vi "Report - Excel.vi"(4 "pdf":bool=TRUE, 5 "Chart Seperation by Order#":bool=TRUE, 6 "Details from .stp and Parameters":string="Transaction Run No\t15\r\nNo.\t1\r\nOrder No.\t105\r\nOper. No.\t1051\r\nQty.\t1052\r\nNCR No.\t1053\r\nCustomer Name\tCustomer 105\r\nProject\tProject 105\r\nSales Order\tSO105\r\nItem No.\tSO105\r\nMaterial\tM105\r\nMaterial Description\tM105 Description\r\nRevision\t\r\nSerial No.\t105\r\nTC1\t2\r\nTC2\t\r\nTC3\t\r\nTC4\t\r\nTC5\t\r\nTC6\t\r\nTC01Plot\t1\r\nTC02Plot\t0\r\nTC03Plot\t0\r\nTC04Plot\t0\r\nTC05Plot\t0\r\nTC06Plot\t0\r\nNotes\t\r\nPermitted Temp Diff\t4\r\nPermitted Time Diff\t30\r\nSequence Number\t1\t2\r\nRamp Rate\t150\t50\r\nTarget Temperature\t60\t40\r\nHold Time Duration\t00:20\t00:00\r\nName\tTemperature Controller\tTemperature Module\tTemperature Module\tTemperature Module\r\nModel\tET-3504\tNI-9211\tNI-9211\tNI-9211\r\nEquipment Serial No.\tE123-02\t12F0001\t12F0002\t12F0003\r\nLast Calibration Date\t2013-12-22\t2014-01-01\t2014-02-02\t2014-09-23\r\nNext Calibration Date\t2014-12-22\t2015-01-01\t2015-09-28\t2015-09-01\r\nEquipment ID\tET-3504 02\tNI-9211 01\tNI-9211 02\tNI-9211 03\r\nNotice Period\t30\t60\t0\t0\r\nWPS/Ref\tWPS2\r\nWPS Rev\t1\r\nHold Temperature\t60\r\nWPS Details Temperature Units\t°C\r\nHold Time (HH:MM)\t00:20\r\nExtra WPS\tWPS2\r\nExtra Rev\t1\r\nAdditional WPS Number\t,\r\nOutput Set\t001\r\nFurnace Serial No\tA1234A1\r\nLast Inspection Date\t2013-12-22\r\nNext Inspection Due Date\t2014-12-22\r\nChannel to Probe Mapping\t1,2,3,4,5,6,7,8,9,10,11,12,13,14,15,16\r\n[StartRecordTime]\t2014-12-02 08:49:30\r\n[StartRecordTemp]\t27.62\r\n[MaxRecordedTemp]\t60.3\r\n[MaxRecordedTempTime]\t2014-12-02 09:04:30\r\n[MinRecordedTemp]\t27.62\r\n[MinRecordedTempTime]\t2014-12-02 08:49:30\r\n[EndRecordTemp]\t37.15\r\n[EndRecordTime]\t2014-12-02 09:50:31\r\n[RecordedMinutes]\t61\r\n[StartHoldTime]\t2014-12-02 09:02:31\r\n[StartHoldTemp]\t60\r\n[HoldTimeMaxTemp]\t60.3\r\n[HoldTimeMinTemp]\t59.75\r\n[EndHoldTime]\t2014-12-02 09:22:31\r\n[EndHoldTemp]\t60\r\n[HoldDurationMinutes]\t0:20\r\n[TempDiffDuringHold]\t0.55\r\n[UnitOfTemperature]\t°C\r\n[PerformedBy]\tadmin\r\n[PerformedOn]\t2014-12-02 08:49:30\r\n[IsTempWithinTol]\t-1\r\n[IsTimeWithinTol]\t-1\r\n[ProcessStatus]\t1\r\n[OverallStatus]\t1\r\n[Result]\t1\r\n[RawDataFilePath]\tc:\\temp\\SRTRS4070_Host\\Data_Host\\2014\\12\\\r\n[RawDataFileName]\t147_20141202_084930.dat\r\n[SavedBy]\tadmin\r\nUsername\tAdministrator\r\n", 7 "Use DB for Picture (Material)":bool=TRUE, 8 "error in (no error)":errorcluster, 9 "Include MetaData":bool=TRUE, 10 "Report Additional Details":T1, 11 "Report Files Cluster":T2) -> (0 "error out":errorcluster, 1 "Picture Error":errorcluster, 2 "Material File":string)   [LabVIEW 2013]
uses:
  Controls/Report Files Cluster.ctl
  Controls/Report Additional Details Cluster.ctl
  Controls/DB - Master Data Material Enum.ctl
  Controls/DB - OpenClose.ctl
  <vilib>/Utility/NIReport.llb/NI_report.lvclass
  <vilib>/Utility/file.llb/Read From Spreadsheet File (string).vi
  Controls/Global SRTRS.vi
  <vilib>/addons/_office/excel.llb/Excel Easy Table (str).vi
  <vilib>/Utility/NIReport.llb/Excel/NI_Excel.lvclass
  <vilib>/addons/_office/NI_ReportGenerationToolkit.lvlib
panel:
  out "DB Error":errorcluster
  in  "Close Excel":bool=TRUE
  in  "Include ConvFromUnicode":bool
  in  "Material":T3
  out "Reference Error Out":errorcluster
  out "Shape Name":string
  out "Order No Data from .dat File":string[][](array[string])
  out "Year":string
  out "Details from .stp and Parameters":string[][](array[string])=[["No.", "2", "", ""], ["Order No.", "123456002", "", ""], ["Operation No.", "202", "", ""], ["Qty (EA)", "201", "", ""], ["NCR No.", "203", "", ""], ["Customer", "Customer 204", "", ""], ["Project", "205", "", ""], ["Sales Order No.", "206", "", ""], ["Item No.", "207", "", ""], ["Material", "102-04", "", ""], ["BOM Rev.", "5", "", ""], ["Material Description", "Mat5", "", ""], ["Serial No.", "208", "", ""], ["TC1", "", "", ""], ["TC2", "", "", ""], ["TC3", "", "", ""], ["TC4", "4", "", ""], ["TC5", "5", "", ""], ["TC6", "6", "", ""], ["Notes", "Notes 200", "", ""], ["User", "Admin", "", ""], ["Customer No.", "", "", ""], ["Sequence Number", "1", "2", ""], ["Ramp Rate (DegC / hour)", "100", "200", ""], ["Target Temperature (DegC)", "200", "400", ""], ["Additional WPS/Ref.", "MyWPS2", "", ""], ["Rev.", "1A", "", ""], ["Module Serial No.", "A12345", "B67890", ""], ["Calibration Date", "2013-11-01", "2013-11-15", ""], ["Calibration Due", "2014-11-01", "2014-11-15", ""], ["WPS/Ref", "MyWPS", "", ""], ["Rev", "1C", "", ""], ["Hold Temperature", "500", "", ""], ["WPS Details Temperature Units", "", "", ""], ["Hold Time (HH:MM)", "4:00", "", ""], ["Furnace Serial No", "100", "", ""], ["Survey Date", "2013-12-05", "", ""], ["Survey Due", "2014-12-05", "", ""]]
  out "pdf file":string="c:\\temp\\SRTRS4070\\Reports\\2013\\0090300212_123456002_20131223_231711.pdf"
  out "abcd.xls":string="0090300212_123456002_20131223_231711.xls"
  out "Month":string="2013"
  out "All Data from .dat File":string[][](array[string])=[["Time", "TC1", "TC2", "TC3", "TC4", "TC5", "TC6", "TC7", "TC8"], ["0", "6.3", "7.3", "7.3", "7.3", "7.3", "7.3", "7.3", "7.3"], ["1", "9.8", "10.8", "10.8", "10.8", "10.8", "10.8", "10.8", "10.8"], ["2", "14.0", "15.0", "15.0", "15.0", "15.0", "15.0", "15.0", "15.0"], ["3", "19.0", "20.0", "20.0", "20.0", "20.0", "20.0", "20.0", "20.0"], ["4", "24.7", "25.7", "25.7", "25.7", "25.7", "25.7", "25.7", "25.7"], ["5", "31.1", "32.1", "32.1", "32.1", "32.1", "32.1", "32.1", "32.1"], ["6", "38.2", "39.2", "39.2", "39.2", "39.2", "39.2", "39.2", "39.2"], ["7", "45.9", "46.9", "46.9", "46.9", "46.9", "46.9", "46.9", "46.9"], ["8", "54.2", "55.2", "55.2", "55.2", "55.2", "55.2", "55.2", "55.2"], ["9", "63.1", "64.1", "64.1", "64.1", "64.1", "64.1", "64.1", "64.1"], ["10", "72.5", "73.5", "73.5", "73.5", "73.5", "73.5", "73.5", "73.5"], ["11", "82.4", "83.4", "83.4", "83.4", "83.4", "83.4", "83.4", "83.4"], ["12", "92.8", "93.8", "93.8", "93.8", "93.8", "93.8", "93.8", "93.8"], ["13", "103.6", "104.7", "104.6", "104.6", "104.7", "104.6", "104.7", "104.6"], ["14", "114.8", "115.8", "115.8", "115.8", "115.8", "115.8", "115.8", "115.8"], ["15", "126.4", "127.4", "127.4", "127.4", "127.4", "127.4", "127.4", "127.4"], ["16", "138.2", "139.2", "139.2", "139.2", "139.2", "139.2", "139.2", "139.2"], ["17", "150.3", "151.3", "151.3", "151.3", "151.3", "151.3", "151.3", "151.3"], ["18", "162.5", "163.5", "163.5", "163.5", "163.5", "163.5", "163.5", "163.5"], ["19", "174.9", "175.9", "175.9", "175.9", "175.9", "175.9", "175.9", "175.9"], ["20", "187.4", "188.4", "188.4", "188.4", "188.4", "188.4", "188.4", "188.4"], ["21", "200.0", "201.0", "201.0", "201.0", "201.0", "201.0", "201.0", "201.0"], ["22", "212.6", "213.6", "213.6", "213.6", "213.6", "213.6", "213.6", "213.6"], ["23", "225.1", "226.1", "226.1", "226.1", "226.1", "226.1", "226.1", "226.1"], ["24", "237.5", "238.5", "238.5", "238.5", "238.5", "238.5", "238.5", "238.5"], ["25", "249.7", "250.7", "250.7", "250.7", "250.7", "250.7", "250.7", "250.7"], ["26", "261.8", "262.8", "262.8", "262.8", "262.8", "262.8", "262.8", "262.8"], ["27", "273.6", "274.6", "274.6", "274.6", "274.6", "274.6", "274.6", "274.6"], ["28", "285.2", "286.2", "286.2", "286.2", "286.2", "286.2", "286.2", "286.2"], ["29", "296.4", "297.3", "297.4", "297.3", "297.4", "297.4", "297.4", "297.3"]]
  # "2014-09-28 19:23"
  # "Transaction No,93\nNo.,2\nOrder No.,102\nOper. No.,102\nQty.,1\nNCR No.,102\nCustomer Name,Cust102\nProject,Proj102\nSales Order,SO102\nItem No.,SOI102\nMaterial,M102\nMaterial Description,Blue Arrow\nRevision,1\nSerial No.,102\nTC1,3\nTC2,4\nTC3,\nTC4,\nTC5,\nTC6,\nTC01Plot,1\nTC02Plot,1\nTC03Plot,0\nTC04Plot,0\nTC05Plot,0\nTC06Plot,0\nNotes,\nSequence Number,1,2\nRamp Rate,200,100\nTarget Temperature,100,25\nHold Time Duration,00:10,00:00\nModule Serial No.,ET-3504,NI-9211,NI-9211,NI-9211\nLast Calibration Date,E12345,12F0531,13C7150,A12345\nNext Calibration Date,2012-11-22,2014-01-01,2014-02-02,2014-09-23\n,2014-11-22,2015-01-01,2015-09-28,2015-09-01\nWPS5\n10\n100\n\n00:10\nWPS5\n10\nFurnace Serial No,A123456\nLast Inspection Date,2012-11-22\nNext Inspection Due Date,2014-11-22\nChannel to Probe Mapping,1,2,3,4,5,6,7,8,9,10,11,12,13,14,15,16\n[StartRecordTime],2014-09-28 19:41:56\n[StartRecordTemp],28.49\n[MaxRecordedTemp],\n[MaxRecordedTempTime],\n[MinRecordedTemp],\n[MinRecordedTempTime],\n[EndRecordTemp],24.89\n[EndRecordTime],2014-09-28 19:43:15\n[RecordedMinutes],-1\n[StartHoldTime],2014-09-28 19:42:18\n[StartHoldTemp],100\n[EndHoldTime],2014-09-28 19:42:28\n[EndHoldTemp],100\n[HoldDurationMinutes],0:00\n[TempDiffDuringHold],-99.5\n[UnitOfTemperature],\n[PerformedBy],100001\n[PerformedOn],2014-09-28 19:41:56\n[IsTempWithinTol],-1\n[IsTimeWithinTol],-1\n[ProcessStatus],P\n[OverallStatus],\n[Result],\n[RawDataFile],\n[RawDataFilePath],c:\\temp\\SRTRS4070_Host\\Data_Host\\2014\\09\n[RawDataFileName],93_20140928_194156.dat"
  # "Error -2146827284\nPossible Causes. \nMicrosoft Excel Refuse to accept ActiveX Client Request\nSolution: \nGoto Task Manager and End Task. \nOr Run cmd line End Task in LabVIEW code"
  # "Error -2146827284\nPossible Causes. \nFile cannot be created\nSolution: \nCheck Access rights to folder"
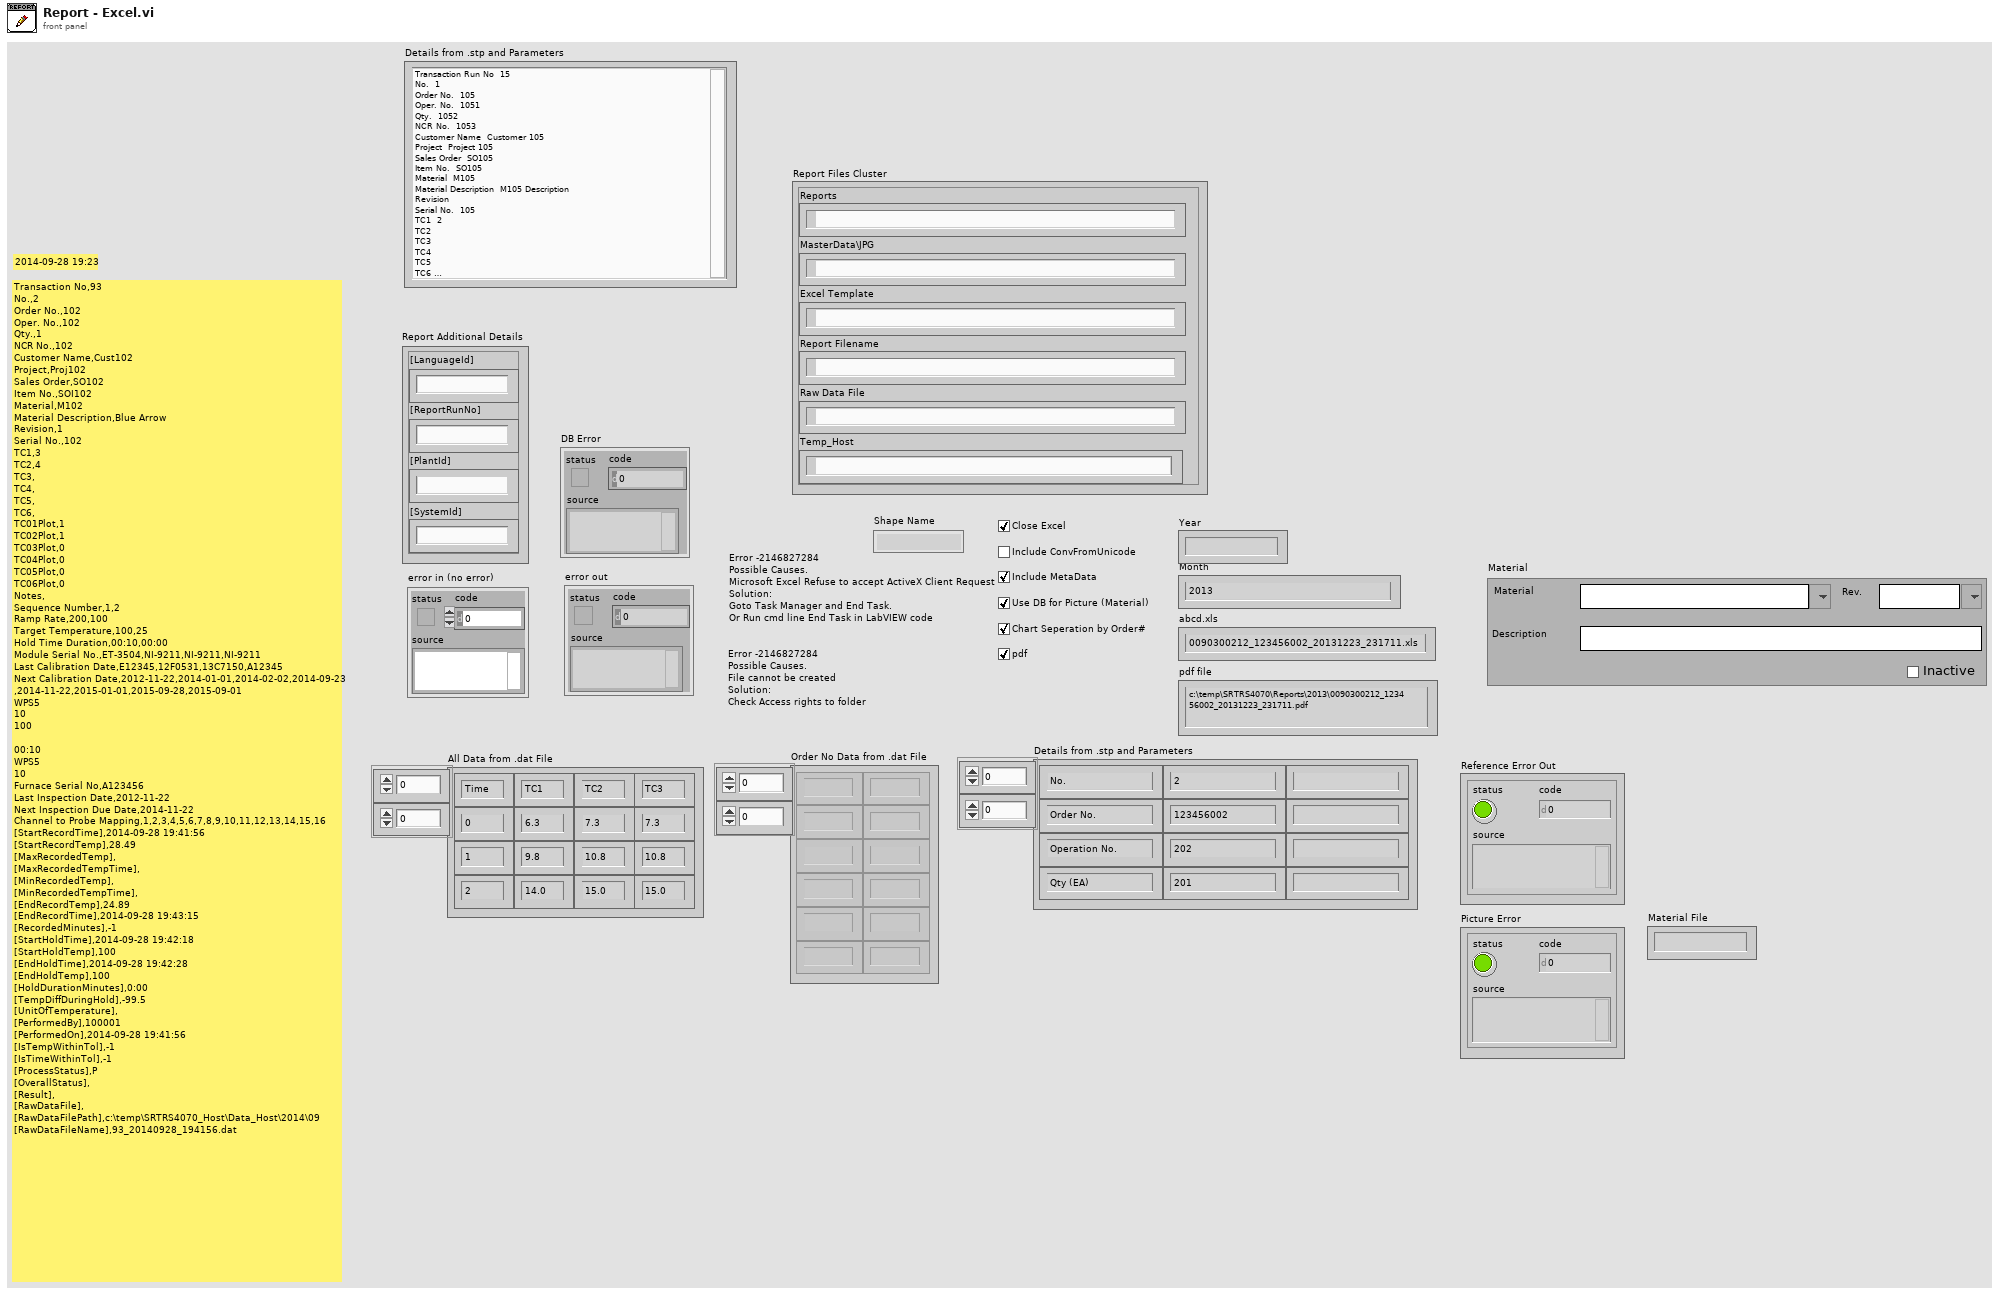
[diagram p1: front panel]
types:
  T1 = typedef "Report Additional Details Cluster.ctl" = cluster{"[LanguageId]":string, "[ReportRunNo]":string, "[PlantId]":string, "[SystemId]":string}
  T2 = typedef "Report Files Cluster.ctl" = cluster{"Reports":path, "MasterData\\JPG":path, "Excel Template":path, "Report Filename":path, "Raw Data File":path, "Temp_Host":path}
  T3 = cluster{"Master Data Material":string, "Master Data Rev":string, "Master Data Material Description":string, "Inactive":bool}
  T4 = cluster{"position (Excel)":cluster{"row":i32, "column":i32}, "name (Excel)":string, "bookmark (Word)":string}
  T5 = enum16{"maximized", "minimized", "normal", "no change"}
  T6 = enum16{"Standard Report", "HTML", "Word", "Excel"}
  T7 = typedef "DB - Logon Extra Info.ctl" = cluster{"Plant Name":string, "UserName":string, "Hostname [ClientName]":string, "IsUnicode":bool}
  T8 = typedef "DB - OpenClose.ctl" = cluster{"Open":bool, "Close":bool}
  T9 = typedef "DB - Master Data Material Enum.ctl" = enum16{"INSERT [MasterData].[Material]", "UPDATE [MasterData].[Material]", "SELECT [MaterialNo]", "SELECT [ShortDescription]", "SELECT [MaterialRev]", "SELECT [Description], [ImageFile]", "SELECT [Description] (Long)"}
  T10 = typedef "NI_Database_API.lvlib/Conn ObjectReference.ctl" = refnum<k1>
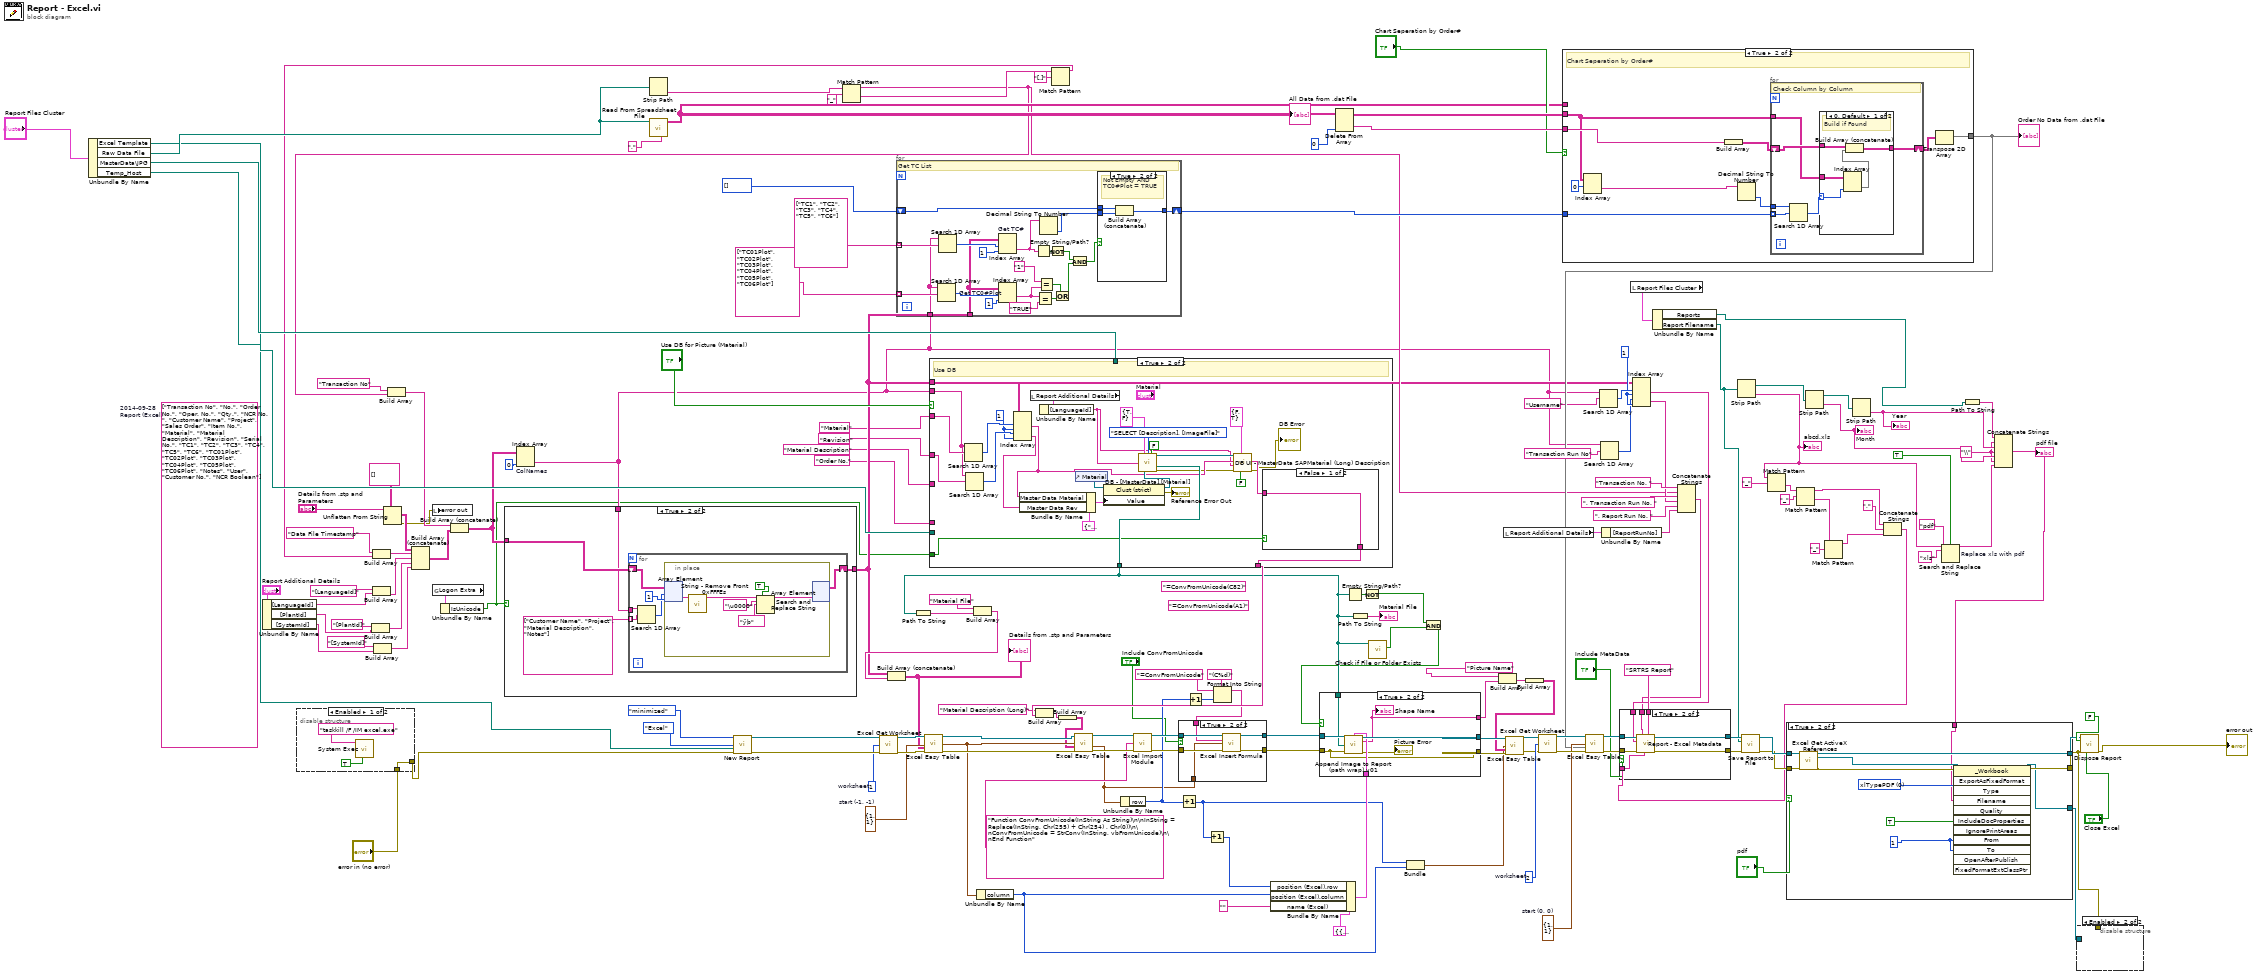
[diagram p0: block diagram]
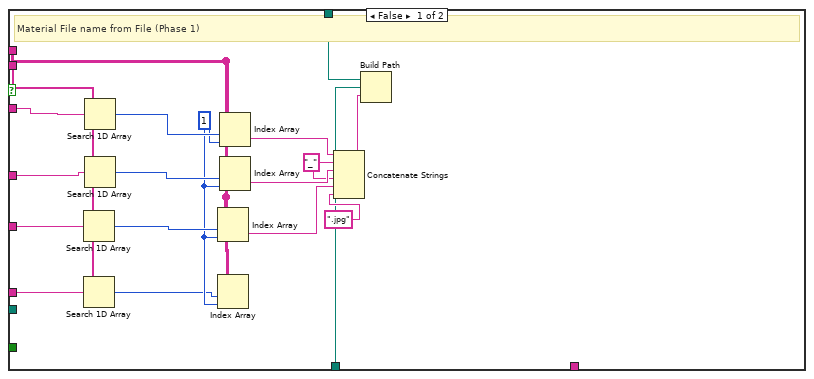
[diagram p5: hidden frame]
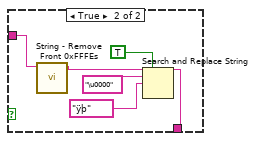
[diagram p6: hidden frame]
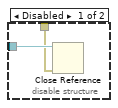
[diagram p11: hidden frame]
diagram:
  (unwired) "=ConvFromUnicode(C82)" ("text")
  (unwired) "=ConvFromUnicode(A1)" ("text")
  (unwired) string[] ["Transaction No", "No.", "Order No.", "Oper. No.", "Qty.", "NCR No.", "Customer Name", "Project", "Sales Order", "Item No.", "Material", "Material Description", "Revision", "Serial No.", "TC1", "TC2", "TC3", "TC4", "TC5", "TC6", "TC01Plot", "TC02Plot", "TC03Plot", "TC04Plot", "TC05Plot", "TC06Plot", "Notes", "User", "Customer No.", "NCR Boolean"]  # 2014-09-28 Report (Excel)
  w107 = 1 ("index (col)")
  w51 = "\\" ("string")
  w157 = cluster{"row":i32, "column":i32} {"row"=1, "column"=1}  # start (0, 0)
  w160 = 2  # worksheet
  w150 = cluster{"row":i32, "column":i32} {"row"=1, "column"=1}  # start (-1, -1)
  w162 = 1  # worksheet
  n1 = Unbundle By Name("Report Files Cluster") -> ("Excel Template"=w70:path, "Raw Data File"=w86:path, "MasterData\\JPG"=w82:path, "Temp_Host"=w81:path)
  n2 = Unbundle By Name("Report Additional Details") -> ("[LanguageId]"=w37:string, "[PlantId]"=w5:string, "[SystemId]"=w3:string)
  n3 = disable-structure shown="Enabled" {
    disable-tunnel: [w166 _] -> w142
    disable-tunnel: "error in (no error)" -> [w166 _]
    frame Enabled {
      n4 = call <vilib>:"System Exec.vi"("run minimized? (F)"=TRUE, "command line"="taskkill /F /IM excel.exe") -> ()  [unwired: 6 in, 4 out]
    }
    frame Disabled {
    }
  }
  n5 = Build Array("[PlantId]" ("string"), w5) -> (w2:string[])
  n6 = Build Array("[LanguageId]" ("string"), w37) -> (w35:string[])
  n7 = Build Array("[SystemId]" ("string"), w3) -> (w1:string[])
  n8 = Unflatten From String(type=string[][] [], binary string="Details from .stp and Parameters") -> (value=w41:string[][], error out=w13:errorcluster)  [unwired: 3 in, 1 out]
  n9 = local write "error out"(w13) -> ()
  n10 = global read "Global SRTRS.vi" "Logon Extra"() -> (w19:T7)
  n11 = Unbundle By Name(w19) -> ("IsUnicode"=w18:bool)
  n12 = Strip Path(path=w86) -> (name=w133:string)  [unwired: 1 out]
  n13 = call-poly <vilib>:"Read From Spreadsheet File.vi"("delimiter (\\t)"="," ("delimiter (\\t)"), "file path (dialog if empty)"=w86) -> ("all rows"=w100:string[][])  [unwired: 5 in, 4 out]
  "All Data from .dat File" <- w100
  n14 = call <vilib>:"New Report.vi"("window state (normal)"=T5."minimized", "report type"=T6."Excel", "template (empty)"=w70, "error in (no error)"=w142) -> ("report out"=w164:refnum<class "NI_report.lvclass">, "error out"=w163:errorcluster)  [unwired: 10 in]
  n15 = Match Pattern(string=w133, regular expression="_") -> (before substring=w33:string, after substring=w131:string)  [unwired: 1 in, 2 out]
  n16 = Build Array("Transaction No" ("string"), w33) -> (w32:string[])
  n17 = call <vilib>:"Excel Get Worksheet.vi"("report in"=w164, "worksheet index (0)"=w162, "error in (no error)"=w163) -> ("report out"=w152:refnum<class "NI_report.lvclass">, "error out"=w151:errorcluster)  [unwired: 11 in]
  n18 = Match Pattern(string=w131, regular expression="[.]") -> (before substring=w39:string)  [unwired: 1 in, 3 out]
  n19 = Build Array("Data File Timestamp" ("string"), w39) -> (w36:string[])
  n20 = Build Array (concatenate)(w41, w36, w35, w2, w1) -> (w31:string[][])
  n21 = Build Array (concatenate)(w32, w31) -> (w29:string[][])
  n22 = Index Array "ColNames"(array=w29, index (col)=0) -> (element=w27:string[])  [unwired: 1 in]
  n23 = case shown="True" w18 {
    tunnel: w29 -> [w168 w172]
    tunnel: [w168 w171] -> w28
    tunnel: w27 -> [_ w170]
    frame False {
      # "Not Unicode, so no 0x00 Bytes"
    }
    frame True {
      n24 = for {
        tunnel: string[] ["Customer Name", "Project", "Material Description", "Notes"] -> [w178] mode=indexing
        tunnel: w170 -> [w177]
        shift-right: [w173] -> w171
        shift-left: w172 -> [w176]
        n25 = Search 1D Array(1D array=w177, element=w178) -> (index of element=w174:i32)  [unwired: 1 in]
        n26 = in-place {
          n27 = in-place-array #1(w176, w174, 1 ("disabled index (col)")) -> (w180:string)
          n28 = call "String - Remove Front 0xFFFEs.vi"("Sting IN"=w180) -> ("String OUT"=w181:string)  [unwired: 10 in]
          n29 = Search and Replace String(replace all?=TRUE ("replace all? (F)"), input string=w181, search string="\u0000", replace string="ÿþ") -> (result string=w179:string)  [unwired: 4 in, 3 out]
          n30 = in-place-array #1(w179) -> (w173:string[][])  [unwired: 2 out]
        }
      }
    }
  }
  n31 = for {
    tunnel: w27 -> [w189]
    tunnel: string[] ["TC1", "TC2", "TC3", "TC4", "TC5", "TC6"] -> [w205] mode=indexing
    tunnel: w28 -> [w194]
    shift-right: [w201] -> w138
    shift-left: i32[] [] -> [w200]
    tunnel: string[] ["TC01Plot", "TC02Plot", "TC03Plot", "TC04Plot", "TC05Plot", "TC06Plot"] -> [w197] mode=indexing
    # "Get TC List"
    n32 = Search 1D Array(1D array=w189, element=w197) -> (index of element=w196:i32)  [unwired: 1 in]
    n33 = Search 1D Array(1D array=w189, element=w205) -> (index of element=w204:i32)  [unwired: 1 in]
    n34 = Index Array "Get TC#"(array=w194, index (row)=w204, index (col)=1) -> (element=w199:string)
    n35 = Index Array "Get TC0#Plot"(array=w194, index (row)=w196, index (col)=1) -> (element=w185:string)
    n36 = Empty String/Path?(string/path=w199) -> (empty?=w202:bool)
    n37 = Equal?(x=w185, y="TRUE") -> (x = y?=w191:bool)
    n38 = Equal?(x="1" ("y"), y=w185) -> (x = y?=w187:bool)
    n39 = Decimal String To Number(string=w199) -> (number=w198:i32)  [unwired: 2 in, 1 out]
    n40 = Not(x=w202) -> (.not. x?=w192:bool)
    n41 = Or(x=w187, y=w191) -> (x .or. y?=w188:bool)
    n42 = And(x=w192, y=w188) -> (x .and. y?=w190:bool)
    n43 = case shown="True" w190 {
      tunnel: w198 -> [_ w209]
      tunnel: [w206 w208] -> w201
      tunnel: w200 -> [w206 w207]
      frame False {
        # "Empty OR\nDo Not Plot"
      }
      frame True {
        # "Not Empty AND\nTC0#Plot = TRUE"
        n44 = Build Array (concatenate)(w207, w209) -> (w208:i32[])
      }
    }
  }
  n45 = case shown="True" "Use DB for Picture (Material)" {
    tunnel: [w219 w249] -> w11
    tunnel: "Material" -> [w218 w248]
    tunnel: "Revision" -> [w217 w244]
    tunnel: "Material Description" -> [w216 _]
    tunnel: w28 -> [w215 w247]
    tunnel: "Order No." -> [w213 _]
    tunnel: w27 -> [w212 w245]
    tunnel: w82 -> [w210 _]
    tunnel: w81 -> [_ _]
    tunnel: [_ w232] -> w66
    tunnel: w18 -> [_ w231]
    frame False {
      w223 = "_" ("string")
      w214 = 1 ("index (col)")
      # "Material File name from File (Phase 1)"
      n46 = Search 1D Array(1D array=w212, element=w216) -> (index of element=w224:i32)  [unwired: 1 in]
      n47 = Search 1D Array(1D array=w212, element=w213) -> (index of element=w211:i32)  [unwired: 1 in]
      n48 = Search 1D Array(1D array=w212, element=w218) -> (index of element=w228:i32)  [unwired: 1 in]
      n49 = Search 1D Array(1D array=w212, element=w217) -> (index of element=w227:i32)  [unwired: 1 in]
      n50 = Index Array(array=w215, index (row)=w224, index (col)=w214) -> (element=w222:string)
      n51 = Index Array(array=w215, index (row)=w211, index (col)=w214) -> ()  [unwired: 1 out]
      n52 = Index Array(array=w215, index (row)=w228, index (col)=w214) -> (element=w226:string)
      n53 = Index Array(array=w215, index (row)=w227, index (col)=w214) -> (element=w225:string)
      n54 = Concatenate Strings(w226, w223, w225, w223, w222, ".jpg" ("string")) -> (w220:string)
      n55 = Build Path(base path=w210, name or relative path=w220) -> (appended path=w219:path)
    }
    frame True {
      w242 = 1 ("disabled index (col)")
      # "Use DB"
      n56 = Search 1D Array(1D array=w245, element=w248) -> (index of element=w246:i32)  [unwired: 1 in]
      n57 = Search 1D Array(1D array=w245, element=w244) -> (index of element=w243:i32)  [unwired: 1 in]
      n58 = Index Array(array=w247, index (row) #1=w246, index (col) #1=w242, index (row) #2=w243, index (col) #2=w242) -> (element #1=w240:string, element #2=w241:string)
      n59 = Bundle By Name(cluster=T3 {"Master Data Material"="", "Master Data Rev"="", "Master Data Material Description"="", "Inactive"=FALSE} ("Value"), "Master Data Material"=w240, "Master Data Rev"=w241) -> (w255:T3)
      n60 = local read "Report Additional Details"() -> (w234:T1)
      n61 = Unbundle By Name(w234) -> ("[LanguageId]"=w233:string)
      n62 = control-ref of="Material"() -> (w251:refnum<vi>)
      n63 = property class="Clust (strict)"(reference=w251, "Value"=w255) -> (reference out=w254:refnum<vi>, error out=→"Reference Error Out":errorcluster)  [unwired: 1 in]
      n64 = call "DB - [MasterData].[Material].vi"("DB Connection"=T8 {"Open"=TRUE, "Close"=FALSE}, "DB - Master Data Material Enum"=DB_-_Master_Data_Material_Enum."SELECT [Description], [ImageFile]", "Include Inactive"=FALSE, "[LanguageId]"=w233, "Clust Refnum"=w254) -> ("connection reference"=w237:T10, "Material File"=w249:path, "SUMMARY"=w235:errorcluster)  [unwired: 6 in, 2 out]
      n65 = call "DB UI - MasterData SAPMaterial (Long) Description.vi"("FP is Modal"=FALSE, "DB Connection"=T8 {"Open"=FALSE, "Close"=TRUE}, "error in (no error)"=w235, "[LanguageId]"=w233, "[MaterialNo]"=w240, "connection reference 2"=w237) -> ("SUMMARY"=→"DB Error":errorcluster, "[Description] (Long)"=w230:string)  [unwired: 3 in, 1 out]
      n66 = case shown="False" w231 {
        tunnel: [w257 w263] -> w232
        tunnel: w230 -> [w257 w259]
        frame False {
        }
        frame True {
          n67 = call "String - Remove Front 0xFFFEs.vi"("Sting IN"=w259) -> ("String OUT"=w258:string)  [unwired: 10 in]
          n68 = Search and Replace String(replace all?=TRUE ("replace all? (F)"), input string=w258, search string="\u0000", replace string="ÿþ") -> (result string=w263:string)  [unwired: 4 in, 3 out]
        }
      }
    }
  }
  n69 = Path To String(path=w11) -> (string=w73:string)
  n70 = Build Array("Material File", w73) -> (w72:string[])
  n71 = Build Array (concatenate)(w28, w72) -> (w129:string[][])
  "Details from .stp and Parameters" <- w129
  n72 = call-poly <vilib>:"Excel Easy Table.vi"("report in"=w152, "start (0, 0)"=w150, "text data"=w129, "error in (no error)"=w151) -> ("report out"=w69:refnum<class "NI_report.lvclass">, "next cell bottom-left"=w64:cluster{"row":i32, "column":i32}, "error out"=w68:errorcluster)  [unwired: 7 in, 2 out]
  n73 = Unbundle By Name(w64) -> ("column"=w67:i32)
  n74 = Build Array("Material Description (Long)", w66) -> (w50:string[])
  n75 = Build Array(w50) -> (w49:string[][])
  n76 = call-poly <vilib>:"Excel Easy Table.vi"("report in"=w69, "start (0, 0)"=w64, "text data"=w49, "error in (no error)"=w68) -> ("report out"=w63:refnum<class "NI_report.lvclass">, "next cell top-right"=w16:cluster{"row":i32, "column":i32}, "error out"=w62:errorcluster)  [unwired: 7 in, 2 out]
  n77 = Unbundle By Name(w16) -> ("row"=w20:i32)
  n78 = call <vilib>:"Excel Import Module.vi"("report in"=w63, "module code (\"\")"="Function ConvFromUnicode(InString As String)\n\nInString = Replace(InString, Chr(255) + Chr(254) , Chr(0))\n\nConvFromUnicode = StrConv(InString, vbFromUnicode)\n\nEnd Function" ("module code (\"\")"), "error in (no error)"=w62) -> ("report out"=w60:refnum<class "NI_report.lvclass">, "error out"=w58:errorcluster)  [unwired: 10 in, 1 out]
  n79 = Increment(x=w20) -> (x+1=w56:i32)
  n80 = Increment(x=w20) -> (x+1=w17:i32)
  n81 = Increment(x=w56) -> (x+1=w90:i32)
  n82 = Format Into String(format string="(C%d)", initial string="=ConvFromUnicode" ("text"), w17) -> (resulting string=w53:string)  [unwired: 1 in, 1 out]
  n83 = case shown="True" "Include ConvFromUnicode" {
    tunnel: w60 -> [w265 w271]
    tunnel: [w265 w270] -> w59
    tunnel: w58 -> [w264 w269]
    tunnel: [w264 w268] -> w57
    tunnel: w53 -> [_ w267]
    tunnel: w16 -> [_ w266]
    frame False {
    }
    frame True {
      n84 = call <vilib>:"Excel Insert Formula.vi"("report in"=w271, "formula"=w267, "start (0, 0)"=w266, "error in (no error)"=w269) -> ("report out"=w270:refnum<class "NI_report.lvclass">, "error out"=w268:errorcluster)  [unwired: 10 in]
    }
  }
  n85 = Bundle By Name(cluster=T4 {"position (Excel)"={"row"=0, "column"=0}, "name (Excel)"="", "bookmark (Word)"=""} ("MS Office parameters"), "position (Excel).row"=w90, "position (Excel).column"=w67, "name (Excel)"="") -> (w141:T4)
  n86 = Delete From Array(array=w100, index (col)=0 ("disabled index (col)")) -> (deleted portion=w136:string[], array with subset deleted=w135:string[][])  [unwired: 2 in]
  n87 = Empty String/Path?(string/path=w11) -> (empty?=w9:bool)
  n88 = Path To String(path=w11) -> (string=→"Material File":string)
  n89 = Not(x=w9) -> (.not. x?=w8:bool)
  n90 = call <vilib>:"Check if File or Folder Exists.vi"("path"=w11) -> ("file or folder exists?"=w10:bool)  [unwired: 8 in, 2 out]
  n91 = Bundle(w56, "column"=w67) -> (w89:cluster{i32, "column":i32})  [unwired: 1 in]
  n92 = And(x=w8, y=w10) -> (x .and. y?=w7:bool)
  n93 = case shown="True" w7 {
    tunnel: w59 -> [w273 w280]
    tunnel: w57 -> [w272 w274]
    tunnel: [w273 w279] -> w98
    tunnel: [w272 w274] -> w96
    tunnel: w141 -> [_ w278]
    tunnel: w11 -> [_ w277]
    tunnel: [_ w276] -> w93
    frame False {
    }
    frame True {
      n94 = call <vilib>:"Append Image to Report (path wrap) v01.vi"("report in"=w280, "MS Office parameters"=w278, "path or URL of image"=w277, "error in (no error)"=w274) -> ("report out"=w279:refnum<class "NI_report.lvclass">, "Shape Name"=w276:string, "error out"=→"Picture Error":errorcluster)  [unwired: 7 in, 2 out]
      "Shape Name" <- w276
    }
  }
  n95 = Build Array("Picture Name", w93) -> (w92:string[])
  n96 = local read "Report Additional Details"() -> (w45:T1)
  n97 = Build Array(w92) -> (w91:string[][])
  n98 = call-poly <vilib>:"Excel Easy Table.vi"("report in"=w98, "start (0, 0)"=w89, "text data"=w91, "error in (no error)"=w96) -> ("report out"=w97:refnum<class "NI_report.lvclass">, "error out"=w95:errorcluster)  [unwired: 7 in, 3 out]
  n99 = call <vilib>:"Excel Get Worksheet.vi"("report in"=w97, "worksheet index (0)"=w160, "error in (no error)"=w95) -> ("report out"=w159:refnum<class "NI_report.lvclass">, "error out"=w158:errorcluster)  [unwired: 11 in]
  n100 = case shown="True" "Chart Seperation by Order#" {
    tunnel: w138 -> [_ w289]
    tunnel: w136 -> [_ w286]
    tunnel: w135 -> [_ w283]
    tunnel: [w281 w282] -> w134
    tunnel: w100 -> [w281 _]
    frame False {
      # "Combine ALL into one Chart. Affects Sheet3 only. All logged TCs will be sent."
    }
    frame True {
      # "Chart Seperation by Order#"
      n101 = Index Array(array=w283, index (row)=0) -> (element=w288:string[])  [unwired: 1 in]
      n102 = Build Array(w286) -> (w285:string[][])
      n103 = Decimal String To Number(string=w288) -> (number=w287:i32[])  [unwired: 2 in, 1 out]
      n104 = for {
        tunnel: w287 -> [w296]
        tunnel: w289 -> [w295] mode=indexing
        shift-right: [w292] -> w284
        shift-left: w285 -> [w293]
        tunnel: w283 -> [w291]
        # "Check Column by Column"
        n105 = Search 1D Array(1D array=w296, element=w295) -> (index of element=w294:i32)  [unwired: 1 in]
        n106 = case shown="0, Default" w294 {
          selector: w294 -> [w298 _]
          tunnel: w293 -> [w301 w302]
          tunnel: w291 -> [w299 _]
          tunnel: [w300 w302] -> w292
          frame 0, Default {
            # "Build if Found"
            n107 = Index Array(array=w299, index (col)=w298) -> (element=w297:string[])  [unwired: 1 in]
            n108 = Build Array (concatenate)(w301, w297) -> (w300:string[][])
          }
          frame -1 {
          }
        }
      }
      n109 = Transpose 2D Array(2D array=w284) -> (transposed array=w282:string[][])
    }
  }
  "Order No Data from .dat File" <- w134
  n110 = call-poly <vilib>:"Excel Easy Table.vi"("report in"=w159, "start (0, 0)"=w157, "text data"=w134, "error in (no error)"=w158) -> ("report out"=w128:refnum<class "NI_report.lvclass">, "error out"=w126:errorcluster)  [unwired: 7 in, 3 out]
  n111 = Search 1D Array(1D array=w27, element="Username") -> (index of element=w110:i32)  [unwired: 1 in]
  n112 = Search 1D Array(1D array=w27, element="Transaction Run No") -> (index of element=w106:i32)  [unwired: 1 in]
  n113 = Unbundle By Name(w45) -> ("[ReportRunNo]"=w44:string)
  n114 = local read "Report Files Cluster"() -> (w85:T2)
  n115 = Index Array(array=w28, index (row) #1=w110, index (col) #1=w107, index (row) #2=w106, index (col) #2=w107) -> (element #1=w109:string, element #2=w103:string)
  n116 = Unbundle By Name(w85) -> ("Reports"=w83:path, "Report Filename"=w84:path)
  n117 = Concatenate Strings("Transaction No. ", w33, ", Transaction Run No. " ("string"), w103, ", Report Run No. " ("string"), w44) -> (w102:string)
  n118 = Strip Path(path=w84) -> (stripped path=w116:path, name=w114:string)
  "abcd.xls" <- w114
  n119 = Match Pattern(string=w114, regular expression="_") -> (after substring=w113:string)  [unwired: 1 in, 3 out]
  n120 = Match Pattern(string=w113, regular expression="_") -> (before substring=w77:string, after substring=w79:string)  [unwired: 1 in, 2 out]
  n121 = Strip Path(path=w116) -> (stripped path=w121:path, name=w124:string)
  "Month" <- w124
  n122 = Match Pattern(string=w79, regular expression="_") -> (before substring=w75:string)  [unwired: 1 in, 3 out]
  n123 = Strip Path(path=w121) -> (name=w123:string)  [unwired: 1 out]
  "Year" <- w123
  n124 = Concatenate Strings(w77, "," ("string"), w75) -> (w74:string)
  n125 = case shown="True" "Include MetaData" {
    tunnel: w128 -> [w304 w312]
    tunnel: [w304 w311] -> w127
    tunnel: w126 -> [w303 w310]
    tunnel: [w303 w309] -> w125
    tunnel: "SRTRS Report" ("title (\"\")") -> [_ w308]
    tunnel: w109 -> [_ w307]
    tunnel: w102 -> [_ w306]
    tunnel: w74 -> [_ w305]
    frame False {
    }
    frame True {
      n126 = call "Report - Excel Metadata.vi"("title (\"\")"=w308, "keywords (\"\")"=w305, "subject (\"\")"=w306, "error in (no error)"=w310, "author (\"\")"=w307, "NI_report in"=w312) -> ("error out"=w309:errorcluster, "NI_report out"=w311:refnum<class "NI_report.lvclass">)  [unwired: 2 in, 2 out]
    }
  }
  n127 = call-dynamic "Save Report to File.vi"("report in"=w127, "report file path"=w84, "error in (no error)"=w125) -> ("report out"=w149:refnum<class "NI_report.lvclass">, "error out"=w148:errorcluster)  [unwired: 11 in]
  n128 = Search and Replace String "Replace xls with pdf"(case sensitive?=TRUE ("ignore case? (F)"), input string=w114, search string="xls", replace string="pdf" ("replace string (\"\")")) -> (result string=w122:string)  [unwired: 4 in, 3 out]
  n129 = Path To String(path=w83) -> (string=w120:string)
  n130 = Concatenate Strings(w120, w51, w123, w51, w124, w51, w122) -> (w115:string)
  "pdf file" <- w115
  n131 = case shown="True" "pdf" {
    tunnel: w149 -> [w314 w323]
    tunnel: [w314 w322] -> w147
    tunnel: w148 -> [w313 w321]
    tunnel: [w313 w320] -> w144
    tunnel: [_ w319] -> w145
    tunnel: w115 -> [_ w315]
    frame False {
    }
    frame True {
      w317 = 1
      w324 = 0 items=["xlTypePDF", "xlTypeXPS"] ("Type")
      n132 = call <vilib>:"Excel Get ActiveX References.vi"("report in"=w323, "error in (no error)"=w321) -> ("report out"=w322:refnum<class "NI_report.lvclass">, "Excel._Workbook"=w325:refnum<k7>, "error out"=w318:errorcluster)  [unwired: 7 in, 4 out]
      n133 = invoke class="_Workbook" method="ExportAsFixedFormat"(reference=w325, error in=w318, "Type"=w324, "Filename"=w315, "IncludeDocProperties"=TRUE, "From"=w317, "To"=w317) -> (reference out=w319:refnum<k7>, error out=w320:errorcluster)  [unwired: 5 in, 10 out]
    }
  }
  n134 = disable-structure shown="Enabled" {
    disable-tunnel: w145 -> [w327 _]
    disable-tunnel: w144 -> [w326 _]
    frame Disabled {
      n135 = Close Reference(reference=w327, error in (no error)=w326) -> ()  [unwired: 1 out]
    }
    frame Enabled {
    }
  }
  n136 = call-dynamic "Dispose Report.vi"("report in"=w147, "wait until printing completed? (T)"=FALSE, "error in (no error)"=w144, "close report? (T)"="Close Excel") -> ("error out"=→"error out":errorcluster)  [unwired: 11 in]
